vi "Evaluate Initial State.vi"(9 "r":dbl=0.2, 10 "Heat Source":T2[](array[typedef])=[{"X"=-0.2, "Y"=-0.4}, {"X"=0.4, "Y"=0.4}], 11 "FEM Grid":T1) -> (3 "Initial":dbl[](array[numeric]))   [LabVIEW 2020, in "Heat Equation Solver.lvlib"]
uses:
  Heat Equation Solver.lvlib
  <vilib>/Utility/miscctls.llb/LVPointDoubleTypeDef.ctl
  FEM Grid.ctl
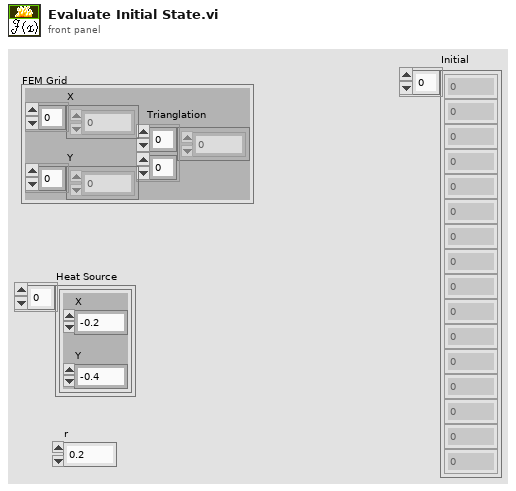
[diagram p1: front panel]
types:
  T1 = typedef "Heat Equation Solver.lvlib/FEM Grid.ctl" = cluster{"X":dbl[], "Y":dbl[], "Trianglation":i32[][]}
  T2 = typedef "LVPointDoubleTypeDef.ctl" = cluster{"X":dbl, "Y":dbl}
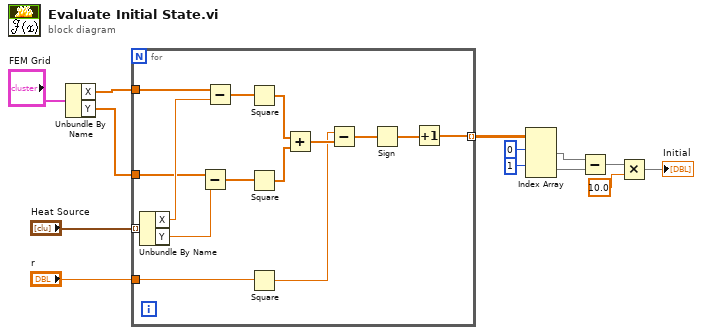
[diagram p0: block diagram]
diagram:
  n1 = Unbundle By Name("FEM Grid") -> ("X"=w2:dbl[], "Y"=w1:dbl[])
  n2 = for {
    tunnel: "Heat Source" -> [w28] mode=indexing
    tunnel: w2 -> [w27]
    tunnel: w1 -> [w25]
    tunnel: [w14] -> w11 mode=indexing
    tunnel: "r" -> [w16]
    n3 = Unbundle By Name(w28) -> ("X"=w26:dbl, "Y"=w24:dbl)
    n4 = Subtract(x=w25, y=w24) -> (x-y=w22:dbl[])
    n5 = Subtract(x=w27, y=w26) -> (x-y=w23:dbl[])
    n6 = Square(x=w23) -> (x^2=w21:dbl[])
    n7 = Square(x=w22) -> (x^2=w20:dbl[])
    n8 = Square(x=w16) -> (x^2=w18:dbl)
    n9 = Add(x=w21, y=w20) -> (x+y=w19:dbl[])
    n10 = Subtract(x=w18, y=w19) -> (x-y=w17:dbl[])
    n11 = Sign(1:w17) -> (0:w15:dbl[])
    n12 = Increment(x=w15) -> (x+1=w14:dbl[])
  }
  n13 = Index Array(array=w11, index (row) #1=0 ("index (row)"), index (row) #2=1 ("index (row)")) -> (element #1=w7:dbl[], element #2=w8:dbl[])  [unwired: 2 in]
  n14 = Subtract(x=w7, y=w8) -> (x-y=w6:dbl[])
  n15 = Multiply(x=w6, y=10.0) -> (x*y=→"Initial":dbl[])
